vi "simulateRobotBehaviour.vi"(8 "error in (no error)":errorcluster, 9 "u_k":dbl[](array[numeric]), 10 "x_k_k":T1, 11 "Game in":refnum<class "Game.lvclass">) -> (0 "error out":errorcluster, 2 "x_k+1":T1, 3 "Game out":refnum<class "Game.lvclass">)   [LabVIEW 2021, in "Game.lvclass"]
uses:
  Game.lvclass
  <vilib>/Analysis/Matrix/Datatypes/RealMatrix.ctl
  <vilib>/Analysis/baseanly.llb/Unit Vector (DBL).vi
  <vilib>/Analysis/baseanly.llb/A x Vector.vi
  <vilib>/Analysis/NI_AALBase.lvlib
  <vilib>/Analysis/Matrix/NI_Matrix.lvlib
panel:
  in  "A":dbl[][](array[numeric])=[[1.0, 0.02, 0.0, 0.0, 2e-05, 0.0, 0.0, 0.0], [0.0, 1.0, 0.0, 0.0, 0.02, 0.0, 0.0, 0.0], [0.0, 0.0, 1.0, 0.02, 0.0, 2e-05, 0.0, 0.0], [0.0, 0.0, 0.0, 1.0, 0.0, 0.02, 0.0, 0.0], [0.0, -50.0, 0.0, 0.0, 0.0, 0.0, 50.0, 0.0], [0.0, 0.0, 0.0, -50.0, 0.0, 0.0, 0.0, 50.0]]
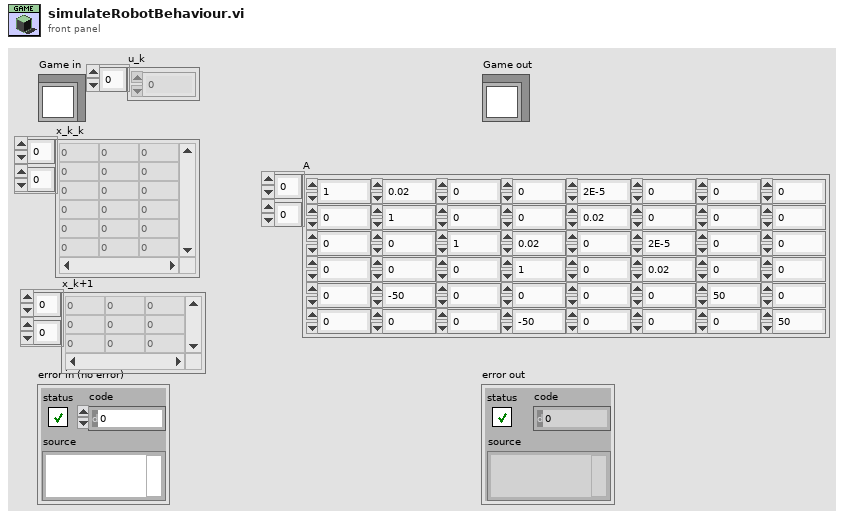
[diagram p1: front panel]
types:
  T1 = typedef "NI_Matrix.lvlib/RealMatrix.ctl" = dbl[][]
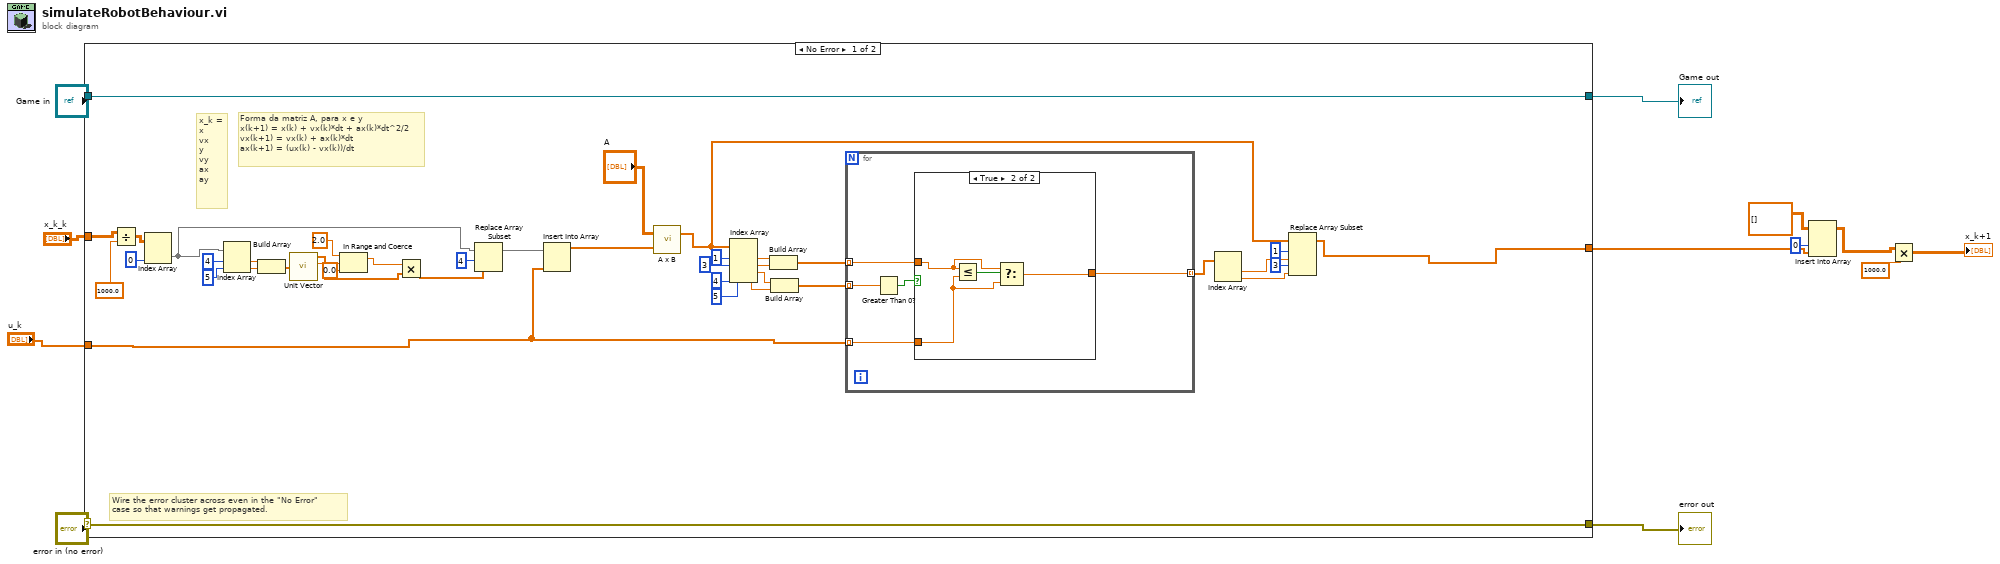
[diagram p0: block diagram]
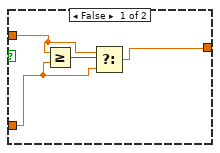
[diagram p2: hidden frame]
diagram:
  n1 = case shown="No Error" "error in (no error)" {
    selector: "error in (no error)" -> [w51 w67]
    tunnel: [w51 w67] -> w11
    tunnel: [w52 w66] -> w9
    tunnel: "Game in" -> [w52 w66]
    tunnel: "u_k" -> [w16 _]
    tunnel: [w36 _] -> w6
    tunnel: "x_k_k" -> [w35 _]
    frame No Error {
      # "Forma da matriz A, para x e y\nx(k+1) = x(k) + vx(k)*dt + ax(k)*dt^2/2\nvx(k+1) = vx(k) + ax(k)*dt\nax(k+1) = (ux(k) - vx(k))/dt"
      # "x_k = \nx \nvx\ny \nvy\nax\nay"
      # "Wire the error cluster across even in the \"No Error\"\ncase so that warnings get propagated."
      n2 = Divide(x=w35, y=1000.0) -> (x/y=w34:T1)
      n3 = Index Array(array=w34, index (col)=0 ("disabled index (col)")) -> (element=w14:dbl[])  [unwired: 1 in]
      n4 = Index Array(array=w14, index #1=4 ("index"), index #2=5 ("index")) -> (element #1=w47:dbl, element #2=w46:dbl)
      n5 = Build Array(w47, w46) -> (w13:dbl[])
      n6 = call-poly <vilib>:"Unit Vector.vi"("Input Vector"=w13) -> ("norm"=w21:dbl, "Unit Vector"=w20:dbl[])  [unwired: 8 in, 1 out]
      n7 = In Range and Coerce(upper limit=2.0, x=w21, lower limit=0.0) -> (coerced(x)=w22:dbl)  [unwired: 1 out]
      n8 = Multiply(x=w22, y=w20) -> (x*y=w19:dbl[])
      n9 = Replace Array Subset(array=w14, new element=w19, index=4) -> (w24:dbl[])
      n10 = Insert Into Array(array=w24, new element=w16) -> (w45:dbl[])  [unwired: 1 in]
      n11 = call-poly <vilib>:"A x B.vi"("Vector"=w45, "A"="A") -> ("A x Vector"=w39:dbl[])  [unwired: 1 out]
      n12 = Index Array(array=w39, index #1=1 ("index"), index #2=3 ("index"), index #3=4 ("index"), index #4=5 ("index")) -> (element #1=w42:dbl, element #2=w41:dbl, element #3=w31:dbl, element #4=w30:dbl)
      n13 = Build Array(w42, w41) -> (w40:dbl[])
      n14 = Build Array(w31, w30) -> (w29:dbl[])
      n15 = for {
        tunnel: w40 -> [w54] mode=indexing
        tunnel: w16 -> [w56] mode=indexing
        tunnel: w29 -> [w55] mode=indexing
        tunnel: [w53] -> w28 mode=indexing
        n16 = Greater Than 0?(x=w55) -> (x > 0?=w57:bool)
        n17 = case shown="True" w57 {
          tunnel: w54 -> [w60 w63]
          tunnel: w56 -> [w59 w62]
          tunnel: [w58 w64] -> w53
          frame False {
            n18 = Greater Or Equal?(x=w60, y=w59) -> (x >= y?=w61:bool)
            n19 = Select(t=w60, s=w61, f=w59) -> (s? t:f=w58:dbl)
          }
          frame True {
            n20 = Less Or Equal?(x=w63, y=w62) -> (x <= y?=w65:bool)
            n21 = Select(t=w63, s=w65, f=w62) -> (s? t:f=w64:dbl)
          }
        }
      }
      n22 = Index Array(array=w28) -> (element #1=w27:dbl, element #2=w26:dbl)  [unwired: 2 in]
      n23 = Replace Array Subset(array=w39, new element #1=w27, index #1=1 ("index"), new element #2=w26, index #2=3 ("index")) -> (w36:dbl[])
    }
    frame Error {
    }
  }
  "error out" <- w11
  "Game out" <- w9
  n24 = Insert Into Array(array=dbl[][] [], index (col)=0 ("disabled index (col)"), new element=w6) -> (w4:dbl[][])  [unwired: 1 in]
  n25 = Multiply(x=w4, y=1000.0) -> (x*y=→"x_k+1":dbl[][])
